vi "Move.vi"(8 "error in (no error)":errorcluster, 10 "targetCoords in":T1, 11 "class data in":refnum<class "Sprite.lvclass">) -> (0 "error out":errorcluster, 3 "class data out":refnum<class "Sprite.lvclass">)   [LabVIEW 2010, in "RenderBase.lvlib" / "Sprite.lvclass"]
doc: "Moves the sprite."
uses:
  Sprite.lvclass
  <vilib>/Utility/miscctls.llb/LV3DPointTypeDef.ctl
  <vilib>/picture/3D Picture Control/NI_3D Picture Control.lvlib
  SceneObject_class/SceneObject.lvclass
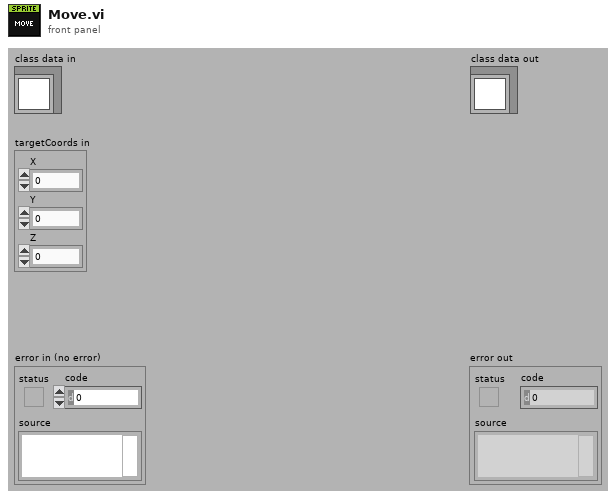
[diagram p1: front panel]
types:
  T1 = typedef "LV3DPointTypeDef.ctl" = cluster{"X":sgl, "Y":sgl, "Z":sgl}
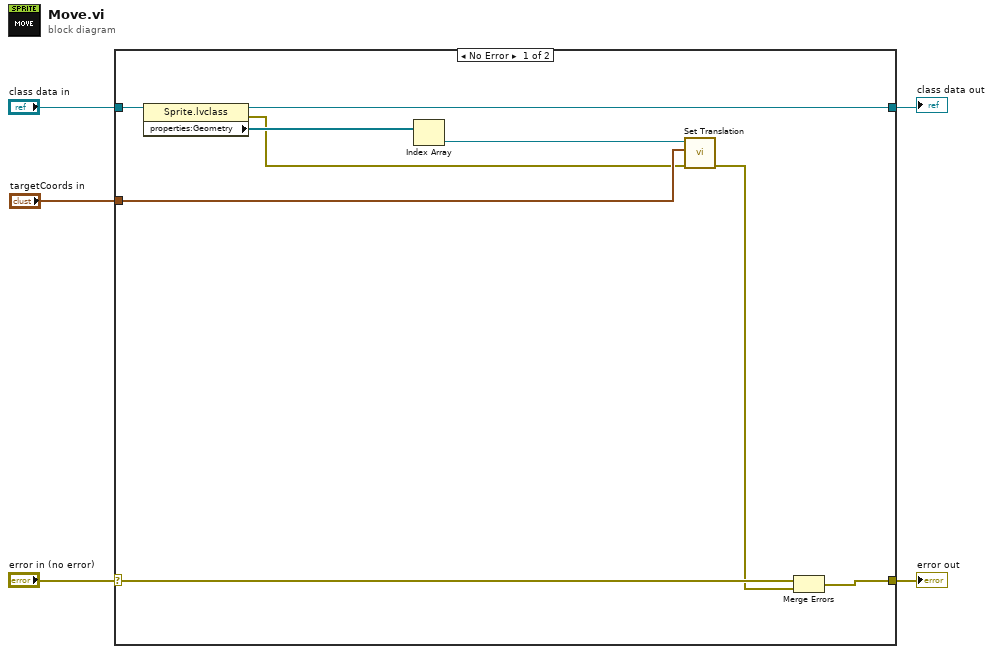
[diagram p0: block diagram]
diagram:
  n1 = case shown="No Error" "error in (no error)" {
    selector: "error in (no error)" -> [w14 w16]
    tunnel: [w8 w16] -> w4
    tunnel: "class data in" -> [w13 w15]
    tunnel: [w12 w15] -> w2
    tunnel: "targetCoords in" -> [w10 _]
    frame No Error {
      n2 = property class="Sprite.lvclass"(reference=w13) -> (reference out=w12:refnum<class "Sprite.lvclass">, error out=w6:errorcluster, "properties:Geometry"=w11:refnum<vi>[])  [unwired: 1 in]
      n3 = Index Array(array=w11) -> (element=w9:refnum<vi>)  [unwired: 1 in]
      n4 = call <vilib>:"Set Translation.vi"("error in (no error)"=w6, "Translation"=w10, "Scene Object"=w9) -> ("error out"=w7:errorcluster)  [unwired: 7 in, 1 out]
      n5 = Merge Errors(w14, w7) -> (w8:errorcluster)
    }
    frame Error {
    }
  }
  "error out" <- w4
  "class data out" <- w2
